vi "ScreenSaverEnabled-Set.vi"(8 "error in (no error)":errorcluster, 10 "Screen Saver Enabled":bool, 11 "Engine in":refnum<class "Engine.lvclass">) -> (0 "error out":errorcluster, 3 "Engine out":refnum<class "Engine.lvclass">)   [LabVIEW 2024, in "GLF.lvlib" / "Engine.lvclass"]
uses:
  Engine.lvclass
  <vilib>/Saukko/LV SDL3/Sources/SDL3/Video/Video.lvlib
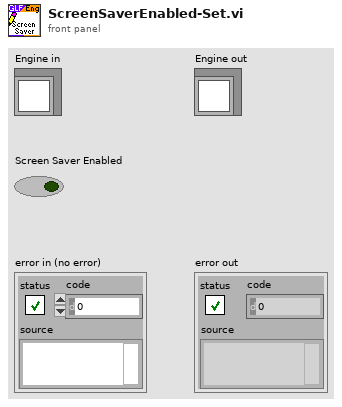
[diagram p1: front panel]
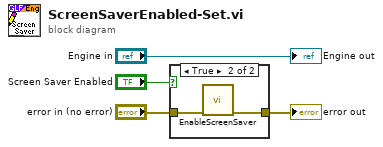
[diagram p0: block diagram]
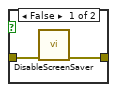
[diagram p2: hidden frame]
diagram:
  n1 = case shown="True" "Screen Saver Enabled" {
    tunnel: "error in (no error)" -> [w6 w8]
    tunnel: [w5 w7] -> w3
    frame False {
      n2 = call <vilib>:"DisableScreenSaver.vi"("No Error"=w6) -> ("Error Out"=w5:errorcluster)  [unwired: 10 in]
    }
    frame True {
      n3 = call <vilib>:"EnableScreenSaver.vi"("No Error"=w8) -> ("Error Out"=w7:errorcluster)  [unwired: 10 in]
    }
  }
  "error out" <- w3
  "Engine out" <- "Engine in"
